vi "test1_160602_75.vi"() -> ()   [LabVIEW 2015]
uses:
  <vilib>/NXT/Block Support/NXT_OutputPort.ctl
  <vilib>/NXT/Block Support/NXT_InputPort.ctl
  <vilib>/NXT/NXTIO Xnodes/NXTIONodeSubVIs/NXTMoveMotors.vi
  <vilib>/NXT/Dual Mode Library/Waits/Wait_Num.vi
  <vilib>/NXT/Dual Mode Library/Sensors/Light_On.vi
  <vilib>/NXT/Dual Mode Library/Sensors/Touch_Pressed.vi
  <vilib>/NXT/Dual Mode Library/Sensors/Sonar_cm.vi
  <vilib>/NXT/NXTIO Xnodes/AddressXNode/NXTIOAddress.xnode
  <vilib>/NXT/Subs/LVHSConnector.ctl
  <vilib>/NXT/NXTIO Xnodes/NXTIOXNode/NXTIO.xnode
  <vilib>/NXT/LegoClasses/BrickReference/BrickReference.lvclass
panel:
  in  "startright/Speed 2":i8=75
  in  "turn lefttC 2":i8=75
  in  "turn lefttB 2":i8=75
  in  "Go-ahead":i8=75
  out "check destance":i16(slide) scale=0.0..100.0
  in  "turn rightC":i8=75
  in  "turn rightB":i8=75
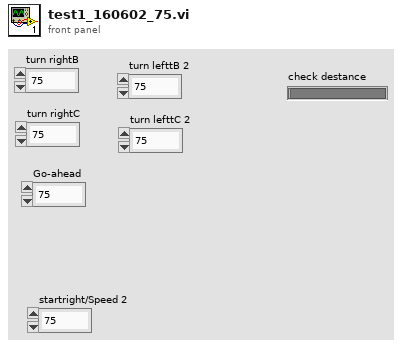
[diagram p1: front panel]
types:
  T1 = typedef "NXT_OutputPort.ctl" = u8
  T2 = typedef "LVHSConnector.ctl" = refnum<class "BrickReference.lvclass">
  T3 = typedef "NXT_InputPort.ctl" = u32
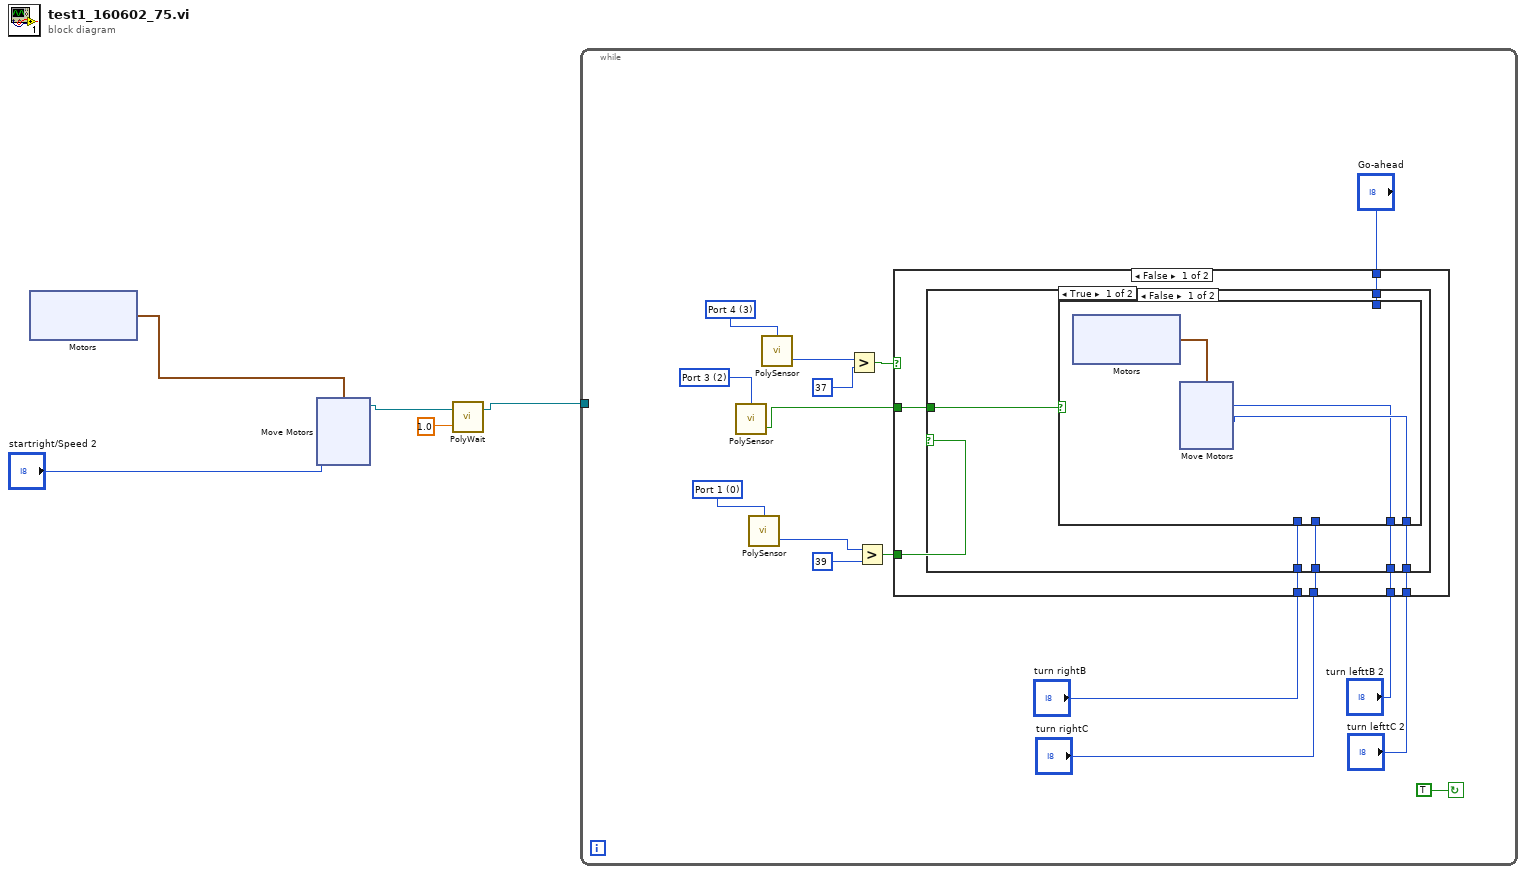
[diagram p0: block diagram]
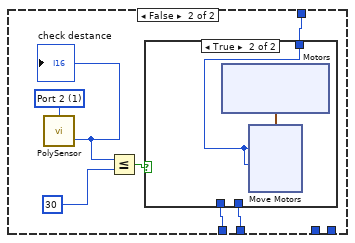
[diagram p2: hidden frame]
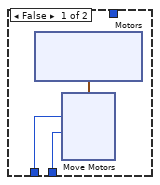
[diagram p3: hidden frame]
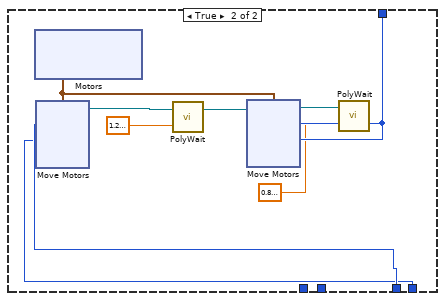
[diagram p4: hidden frame]
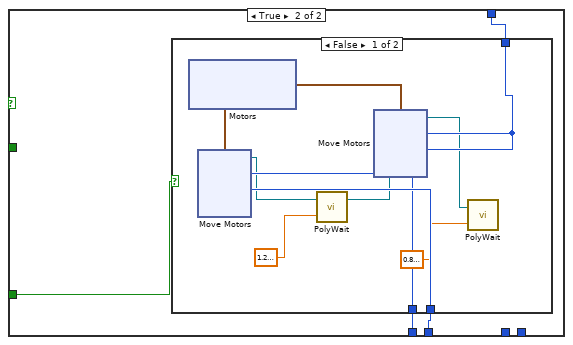
[diagram p5: hidden frame]
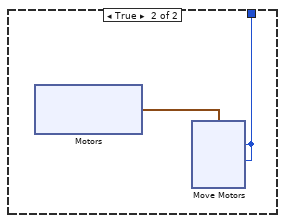
[diagram p6: hidden frame]
diagram:
  n1 = xnode "Motors"() -> ("Motor"=w5:cluster{"Port":T1, "Port":T1})
  n2 = xnode "Move Motors"("Power/Speed 1"="startright/Speed 2", "Motors"=w5, "Power/Speed 2"="startright/Speed 2") -> ("NXT/EV3"=w4:T2)  [unwired: 1 in]
  n3 = call-poly <vilib>:"PolyWait.vi"("Time (1 sec)"=sgl 1.0, "NXT/EV3"=w4) -> ("NXT/EV3"=w3:T2)  [unwired: 2 in]
  n4 = while {
    tunnel: w3 -> [_]
    stop <- TRUE continue-if-true
    w6 = T3 2 items=["Port 1", "Port 2", "Port 3", "Port 4"] ("Port (Port 1)")
    w17 = T3 3 items=["Port 1", "Port 2", "Port 3", "Port 4"] ("Port (Port 3)")
    w16 = T3 0 items=["Port 1", "Port 2", "Port 3", "Port 4"] ("Port (Port 3)")
    n5 = call-poly <vilib>:"PolySensor.vi"("Port (Port 1)"=w6) -> ("Yes / No"=w7:bool)  [unwired: 2 in, 1 out]
    n6 = call-poly <vilib>:"PolySensor.vi"("Port (Port 3)"=w16) -> ("Scaled Value"=w18:i16)  [unwired: 2 in, 1 out]
    n7 = call-poly <vilib>:"PolySensor.vi"("Port (Port 3)"=w17) -> ("Scaled Value"=w20:i16)  [unwired: 2 in, 1 out]
    n8 = Greater?(x=w20, y=i16 37) -> (0:w15:bool)
    n9 = Greater?(x=w18, y=i16 39) -> (0:w14:bool)
    n10 = case shown="False" w15 {
      tunnel: w14 -> [w28 w106]
      tunnel: "turn rightB" -> [w27 w105]
      tunnel: "turn rightC" -> [w26 w104]
      tunnel: "Go-ahead" -> [w25 w103]
      tunnel: "turn lefttB 2" -> [w24 _]
      tunnel: "turn lefttC 2" -> [w23 _]
      tunnel: w7 -> [w22 _]
      frame False {
        n11 = case shown="False" w28 {
          tunnel: w27 -> [w34 _]
          tunnel: w26 -> [w33 _]
          tunnel: w25 -> [w32 w81]
          tunnel: w24 -> [w30 w85]
          tunnel: w23 -> [w29 w84]
          tunnel: w22 -> [w31 _]
          frame False {
            n12 = case shown="True" w31 {
              tunnel: w34 -> [_ w53]
              tunnel: w33 -> [_ w52]
              tunnel: w32 -> [_ w47]
              tunnel: w30 -> [w35 _]
              tunnel: w29 -> [w36 _]
              frame True {
                n13 = xnode "Motors"() -> ("Motor"=w37:cluster{"Port":T1, "Port":T1})
                n14 = xnode "Move Motors"("Power/Speed 2"=w36, "Power/Speed 1"=w35, "Motors"=w37) -> ()  [unwired: 1 in, 1 out]
              }
              frame False {
                w50 = T3 1 items=["Port 1", "Port 2", "Port 3", "Port 4"] ("Port (Port 4)")
                n15 = call-poly <vilib>:"PolySensor.vi"("Port (Port 4)"=w50) -> ("Distance (cm)"=w51:i16)  [unwired: 2 in, 1 out]
                "check destance" <- w51
                n16 = Less Or Equal?(x=w51, y=i16 30) -> (x <= y?=w48:bool)
                n17 = case shown="True" w48 {
                  tunnel: w53 -> [w55 _]
                  tunnel: w52 -> [w54 _]
                  tunnel: w47 -> [_ w66]
                  frame False {
                    n18 = xnode "Motors"() -> ("Motor"=w56:cluster{"Port":T1, "Port":T1})
                    n19 = xnode "Move Motors"("Power/Speed 2"=w54, "Power/Speed 1"=w55, "Motors"=w56) -> ()  [unwired: 1 in, 1 out]
                  }
                  frame True {
                    n20 = xnode "Motors"() -> ("Motor"=w67:cluster{"Port":T1, "Port":T1})
                    n21 = xnode "Move Motors"("Power/Speed 2"=w66, "Power/Speed 1"=w66, "Motors"=w67) -> ()  [unwired: 1 in, 1 out]
                  }
                }
              }
            }
          }
          frame True {
            n22 = xnode "Motors"() -> ("Motor"=w82:cluster{"Port":T1, "Port":T1})
            n23 = xnode "Move Motors"("Power/Speed 2"=w84, "Power/Speed 1"=w85, "Motors"=w82) -> ("NXT/EV3"=w83:T2)  [unwired: 1 in]
            n24 = call-poly <vilib>:"PolyWait.vi"("Time (1 sec)"=sgl 1.3, "NXT/EV3"=w83) -> ("NXT/EV3"=w80:T2)  [unwired: 2 in]
            n25 = xnode "Move Motors"("Power/Speed 2"=w81, "Power/Speed 1"=w81, "Motors"=w82, "NXT/EV3"=w80) -> ("NXT/EV3"=w79:T2)
            n26 = call-poly <vilib>:"PolyWait.vi"("Time (1 sec)"=sgl 0.8, "NXT/EV3"=w79) -> ()  [unwired: 2 in, 1 out]
          }
        }
      }
      frame True {
        n27 = case shown="False" w106 {
          tunnel: w105 -> [w114 _]
          tunnel: w104 -> [w115 _]
          tunnel: w103 -> [w112 w133]
          frame False {
            n28 = xnode "Motors"() -> ("Motor"=w113:cluster{"Port":T1, "Port":T1})
            n29 = xnode "Move Motors"("Power/Speed 2"=w115, "Power/Speed 1"=w114, "Motors"=w113) -> ("NXT/EV3"=w111:T2)  [unwired: 1 in]
            n30 = call-poly <vilib>:"PolyWait.vi"("Time (1 sec)"=sgl 1.3, "NXT/EV3"=w111) -> ("NXT/EV3"=w110:T2)  [unwired: 2 in]
            n31 = xnode "Move Motors"("Power/Speed 2"=w112, "Power/Speed 1"=w112, "Motors"=w113, "NXT/EV3"=w110) -> ("NXT/EV3"=w109:T2)
            n32 = call-poly <vilib>:"PolyWait.vi"("Time (1 sec)"=sgl 0.8, "NXT/EV3"=w109) -> ()  [unwired: 2 in, 1 out]
          }
          frame True {
            n33 = xnode "Motors"() -> ("Motor"=w134:cluster{"Port":T1, "Port":T1})
            n34 = xnode "Move Motors"("Power/Speed 2"=w133, "Power/Speed 1"=w133, "Motors"=w134) -> ()  [unwired: 1 in, 1 out]
          }
        }
      }
    }
  }
